vi "Process LC Data.vi"(1 "LC Indicator Cluster":T1, 2 "Array":dbl[](array[numeric])) -> (0 "PS Data Cluster":T2 {"LC 4" scale=0.0..10.0; "LC 3" scale=0.0..10.0; "LC 2" scale=0.0..10.0; "LC 1" scale=0.0..10.0})   [LabVIEW 2017]
uses:
  Controls/LC Indicator Cluster.ctl
  Controls/LC Calibration Cluster.ctl
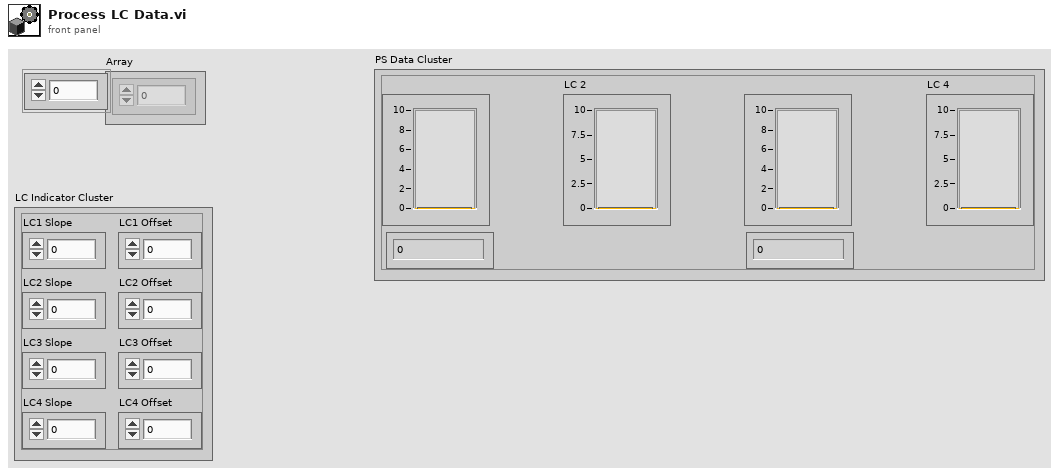
[diagram p1: front panel]
types:
  T1 = typedef "LC Calibration Cluster.ctl" = cluster{"LC1 Slope":dbl, "LC1 Offset":dbl, "LC2 Slope":dbl, "LC2 Offset":dbl, "LC3 Slope":dbl, "LC3 Offset":dbl, "LC4 Slope":dbl, "LC4 Offset":dbl}
  T2 = typedef "LC Indicator Cluster.ctl" = cluster{"LC 1":dbl, "LC 2":dbl, "LC 3":dbl, "LC 4":dbl}
  T3 = cluster{"[0]":dbl, "[1]":dbl, "[2]":dbl, "[3]":dbl, "[4]":dbl, "[5]":dbl, "[6]":dbl, "[7]":dbl, "[8]":dbl}
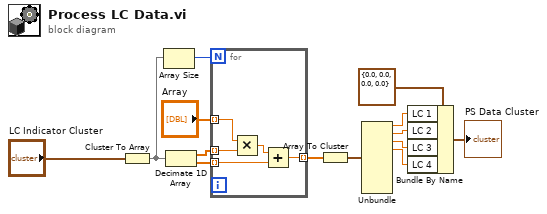
[diagram p0: block diagram]
diagram:
  n1 = Cluster To Array(cluster="LC Indicator Cluster") -> (array=w11:dbl[])
  n2 = Array Size(array=w11) -> (size(s)=w12:i32)
  n3 = Decimate 1D Array(w11) -> (w13:dbl[], w14:dbl[])
  n4 = for {
    N: w12 -> [_]
    tunnel: w14 -> [w16] mode=indexing
    tunnel: w13 -> [w15] mode=indexing
    tunnel: "Array" -> [w19] mode=indexing
    tunnel: [w17] -> w8 mode=indexing
    n5 = Multiply(x=w19, y=w15) -> (x*y=w18:dbl)
    n6 = Add(x=w18, y=w16) -> (x+y=w17:dbl)
  }
  n7 = Array To Cluster(array=w8) -> (cluster=w7:T3)
  n8 = Unbundle(w7) -> ("[0]"=w4:dbl, "[1]"=w3:dbl, "[2]"=w2:dbl, "[3]"=w1:dbl)  [unwired: 5 out]
  n9 = Bundle By Name(cluster=T2 {"LC 1"=0.0, "LC 2"=0.0, "LC 3"=0.0, "LC 4"=0.0} ("PS Data Cluster"), "LC 1"=w4, "LC 2"=w3, "LC 3"=w2, "LC 4"=w1) -> (→"PS Data Cluster":T2)
